vi "Get Y Axis Name.vi"(4 "gain units":T1 caption="Gain", 6 "THD units":T1 caption="THD", 8 "THD+N units":T1 caption="THD+N", 9 "SNR units":T2 caption="SNR", 11 "y-axis data":T3 caption="Y-axis") -> (3 "units":string)   [LabVIEW 2021, in "Efficiency Sweep_Class D Amplifier_UI.lvlib"]
uses:
  Efficiency Sweep_Class D Amplifier_UI.lvlib
  Y axis data selection.ctl
  shared/controls/units - snr.ctl
  shared/controls/units - ratio.ctl
  shared/controls/audio controls.lvlib
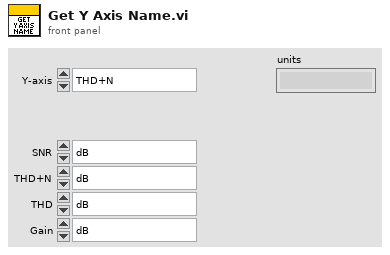
[diagram p1: front panel]
types:
  T1 = typedef "audio controls.lvlib/units - ratio.ctl" = enum32{"dB", "%", "x/y"}
  T2 = typedef "audio controls.lvlib/units - snr.ctl" = enum32{"dB", "x/y"}
  T3 = typedef "Efficiency Sweep_Class D Amplifier_UI.lvlib/Y axis data selection.ctl" = enum32{"THD+N", "THD", "SNR", "Gain", "Amplitude (dBFS)", "Amplitude (Vrms)", "Output Power (W)", "Dynamic Range (dB)", "SFDR (dBc)"}
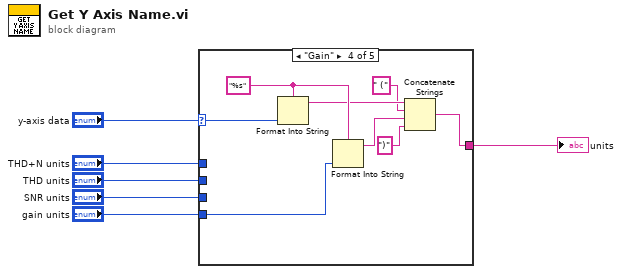
[diagram p0: block diagram]
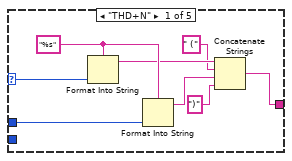
[diagram p2: hidden frame]
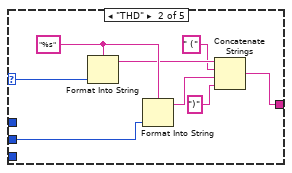
[diagram p3: hidden frame]
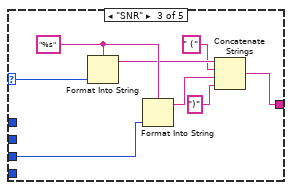
[diagram p4: hidden frame]
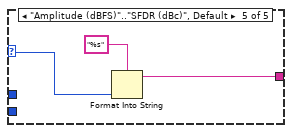
[diagram p5: hidden frame]
diagram:
  n1 = case shown="\"Gain\"" "y-axis data" {
    selector: "y-axis data" -> [w13 w22 w30 w38 w40]
    tunnel: "THD+N units" -> [w14 _ _ _ _]
    tunnel: "THD units" -> [_ w15 _ _ _]
    tunnel: "SNR units" -> [_ _ w23 _ _]
    tunnel: "gain units" -> [_ _ _ w31 _]
    tunnel: [w9 w18 w26 w34 w39] -> w1
    frame "THD+N" {
      w12 = "%s" ("format string")
      n2 = Format Into String(format string=w12, w13) -> (resulting string=w11:string)  [unwired: 2 in, 1 out]
      n3 = Format Into String(format string=w12, w14) -> (resulting string=w10:string)  [unwired: 2 in, 1 out]
      n4 = Concatenate Strings(w11, " (" ("string"), w10, ")" ("string")) -> (w9:string)
    }
    frame "THD" {
      w21 = "%s" ("format string")
      n5 = Format Into String(format string=w21, w22) -> (resulting string=w20:string)  [unwired: 2 in, 1 out]
      n6 = Format Into String(format string=w21, w15) -> (resulting string=w19:string)  [unwired: 2 in, 1 out]
      n7 = Concatenate Strings(w20, " (" ("string"), w19, ")" ("string")) -> (w18:string)
    }
    frame "SNR" {
      w29 = "%s" ("format string")
      n8 = Format Into String(format string=w29, w30) -> (resulting string=w28:string)  [unwired: 2 in, 1 out]
      n9 = Format Into String(format string=w29, w23) -> (resulting string=w27:string)  [unwired: 2 in, 1 out]
      n10 = Concatenate Strings(w28, " (" ("string"), w27, ")" ("string")) -> (w26:string)
    }
    frame "Gain" {
      w37 = "%s" ("format string")
      n11 = Format Into String(format string=w37, w38) -> (resulting string=w36:string)  [unwired: 2 in, 1 out]
      n12 = Format Into String(format string=w37, w31) -> (resulting string=w35:string)  [unwired: 2 in, 1 out]
      n13 = Concatenate Strings(w36, " (" ("string"), w35, ")" ("string")) -> (w34:string)
    }
    frame "Amplitude (dBFS)".."SFDR (dBc)", Default {
      n14 = Format Into String(format string="%s", w40) -> (resulting string=w39:string)  [unwired: 2 in, 1 out]
    }
  }
  "units" <- w1
